vi "Controller.vi"(8 "error in (no error)":errorcluster) -> (0 "error out":errorcluster)   [LabVIEW 2017]
uses:
  Type Definitions/Controller Data.ctl
  Type Definitions/DB Data.ctl
  Type Definitions/DB Info.ctl
  Type Definitions/Display Data.ctl
  Type Definitions/DB Record.ctl
  Type Definitions/Display Console States.ctl
  Type Definitions/GUI Data.ctl
  Type Definitions/Controller States.ctl
  Type Definitions/Sensor UI Data.ctl
  Type Definitions/Queue FG Options.ctl
  Type Definitions/Display Console Message.ctl
  Type Definitions/Sensor Message.ctl
  Type Definitions/Sensor States.ctl
  Type Definitions/GUI Message.ctl
  Type Definitions/Database States.ctl
  Type Definitions/Database Message.ctl
  Type Definitions/Timer States.ctl
  Type Definitions/Controller Message.ctl
  Current State.vi
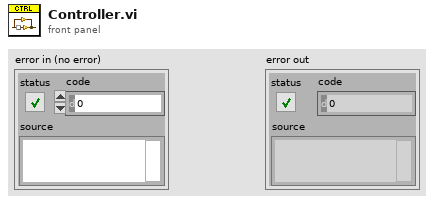
[diagram p1: front panel]
types:
  T1 = typedef "Controller Data.ctl" = cluster{"Time":dbl, "DB Data in":T2, "Display Data":T4, "GUI Data ":T7, "Sensor UI":T9, "Controller States":T8}
  T2 = typedef "DB Data.ctl" = cluster{"Account":i32, "First Name":string, "Last Name":string, "Balance":fxp<+/-,64,35>, "DB Info":T3}
  T3 = typedef "DB Info.ctl" = enum16{"Empty", "Verify", "Login Accepted", "Invalid Login", "Deposit Complete", "Withdrawal Complete", "Withdrawal Failed", "Terminate"}
  T4 = typedef "Display Data.ctl" = cluster{"Message Text":string, "DB Record":T5, "Card Read":bool, "Display Console States":T6}
  T5 = typedef "DB Record.ctl" = cluster{"Account":i32, "First Name":string, "Last Name":string, "Balance":fxp<+/-,64,35>}
  T6 = typedef "Display Console States.ctl" = enum16{"Timeout", "Initial", "Login", "Invalid Login", "Idle", "Balance Inquiry", "Deposit", "Withdrawal", "Fast Cash", "Withdrawal Failed", "Withdrawal Complete", "Terminate", "Shutdown"}
  T7 = typedef "GUI Data.ctl" = cluster{"Card Reader":enum8{"Enabled", "Disabled", "Disabled and Grayed Out"}, "Keypad":enum8{"Enabled", "Disabled", "Disabled and Grayed Out"}, "Balance Inquiry":enum8{"Enabled", "Disabled", "Disabled and Grayed Out"}, "Deposit":enum8{"Enabled", "Disabled", "Disabled and Grayed Out"}, "Withdrawal":enum8{"Enabled", "Disabled", "Disabled and Grayed Out"}, "Fast Cash":enum8{"Enabled", "Disabled", "Disabled and Grayed Out"}, "New Transaction":enum8{"Enabled", "Disabled", "Disabled and Grayed Out"}, "Terminate Session":enum8{"Enabled", "Disabled", "Disabled and Grayed Out"}, "Pinpad Value":string, "Timeout":i32, "Controller States":T8}
  T8 = typedef "Controller States.ctl" = enum16{"Timeout", "Initial", "Login", "Idle", "Balance Inquiry", "Deposit", "Withdrawal", "Fast Cash", "Terminate", "Wait on Exit", "Shutdown", "Error Handler"}
  T9 = typedef "Sensor UI Data.ctl" = cluster{"Funds dispensed":enum16{"Enabled", "Disabled", "Disabled and Grayed Out"}, "Deposit received":enum16{"Enabled", "Disabled", "Disabled and Grayed Out"}, "Timeout":dbl}
  T10 = typedef "Queue FG Options.ctl" = enum16{"Set", "Get", "Read", "Write", "Destroy"}
  T11 = enum8{"Enabled", "Disabled", "Disabled and Grayed Out"}
  T12 = typedef "GUI Message.ctl" = cluster{"Message Info":T8, "Message Data":variant}
  T13 = enum16{"Enabled", "Disabled", "Disabled and Grayed Out"}
  T14 = typedef "Sensor States.ctl" = enum16{"Initial", "Idle", "Shutdown"}
  T15 = typedef "Sensor Message.ctl" = cluster{"Message Info":T14, "Message Data":variant}
  T16 = typedef "Display Console Message.ctl" = cluster{"Message Info":T6, "Message Data":variant}
  T17 = typedef "Database Message.ctl" = cluster{"Message Info":T18, "Message Data":variant}
  T18 = typedef "Database States.ctl" = enum16{"Initial", "Verify", "Balance Inquiry", "Deposit", "Withdrawal", "Fast Cash", "Terminate", "Shutdown"}
  T19 = typedef "Timer States.ctl" = enum16{"Set", "Get"}
  T20 = typedef "Controller Message.ctl" = cluster{"Message Info":T8, "Message Data":variant}
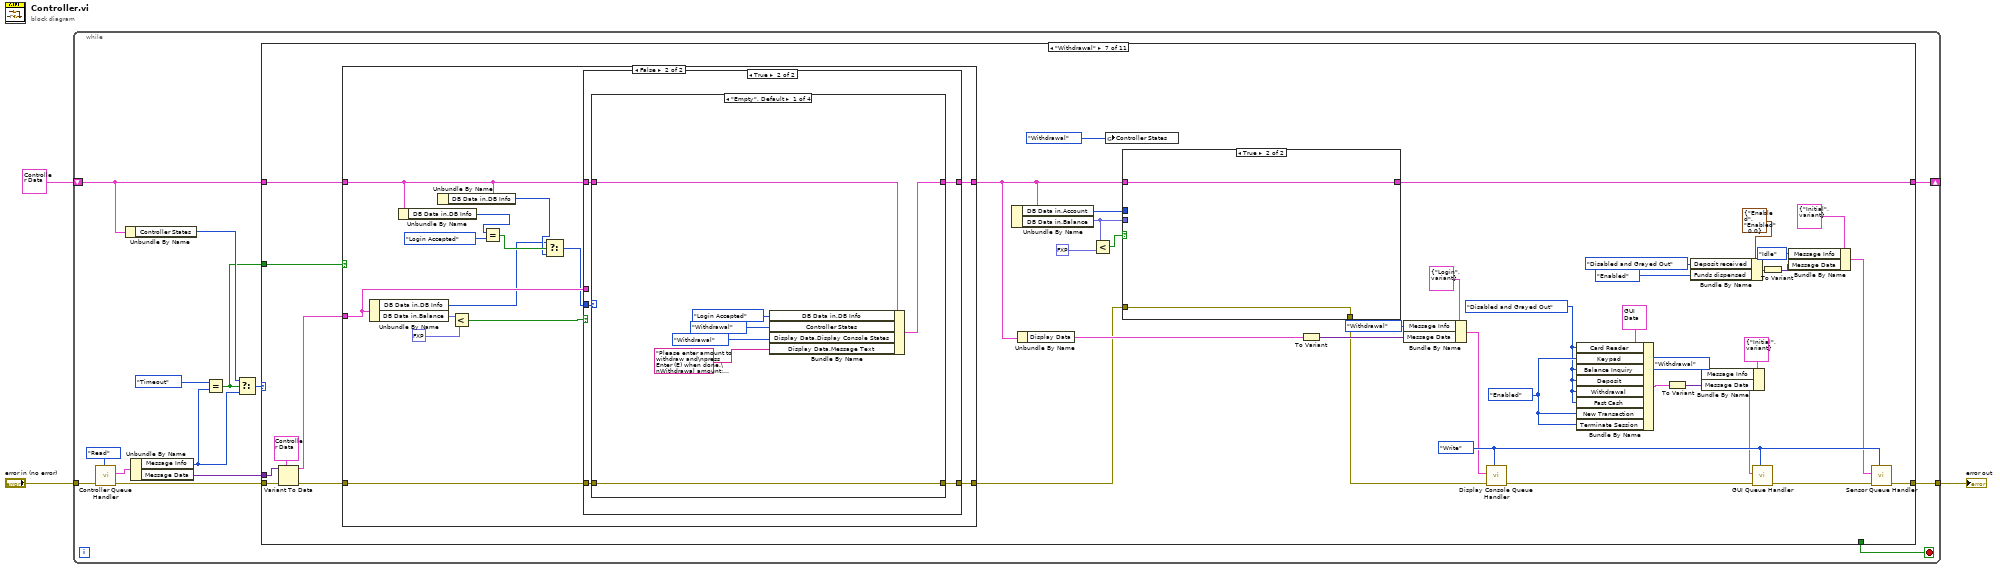
[diagram p0: block diagram]
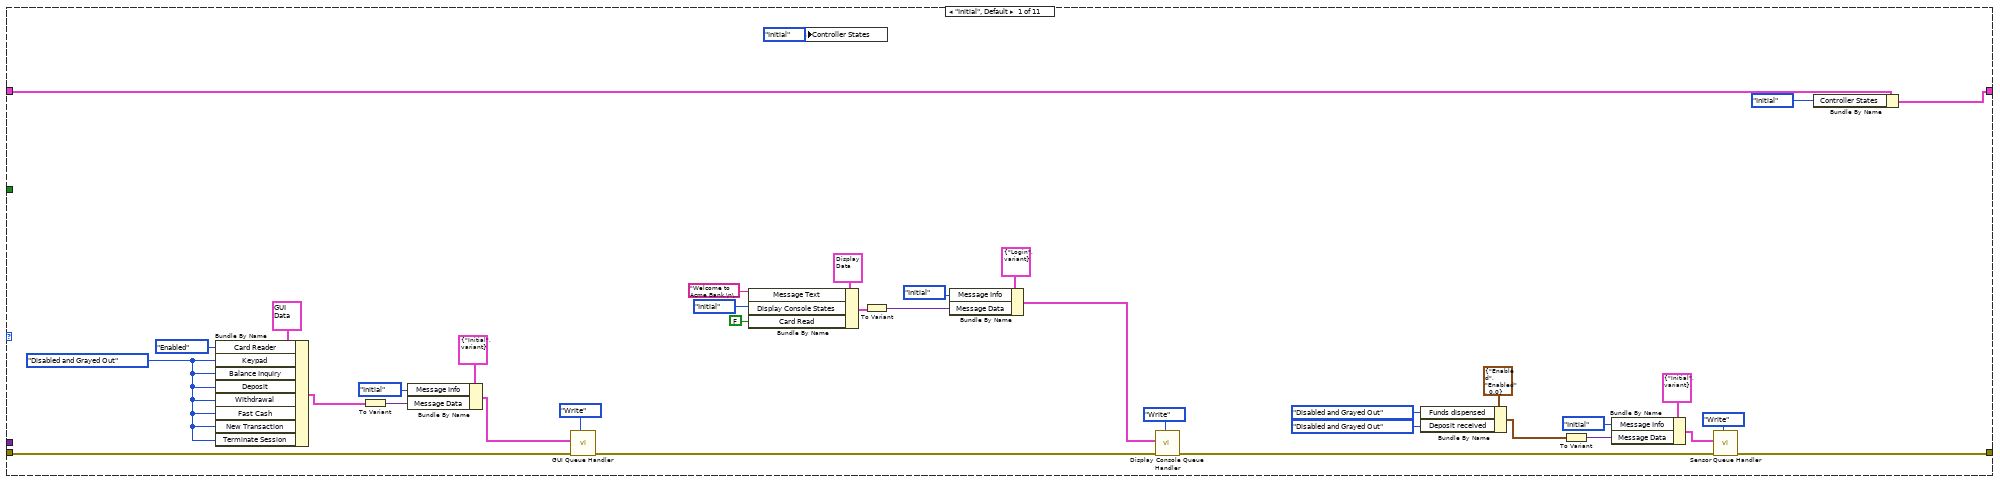
[diagram p2: hidden frame]
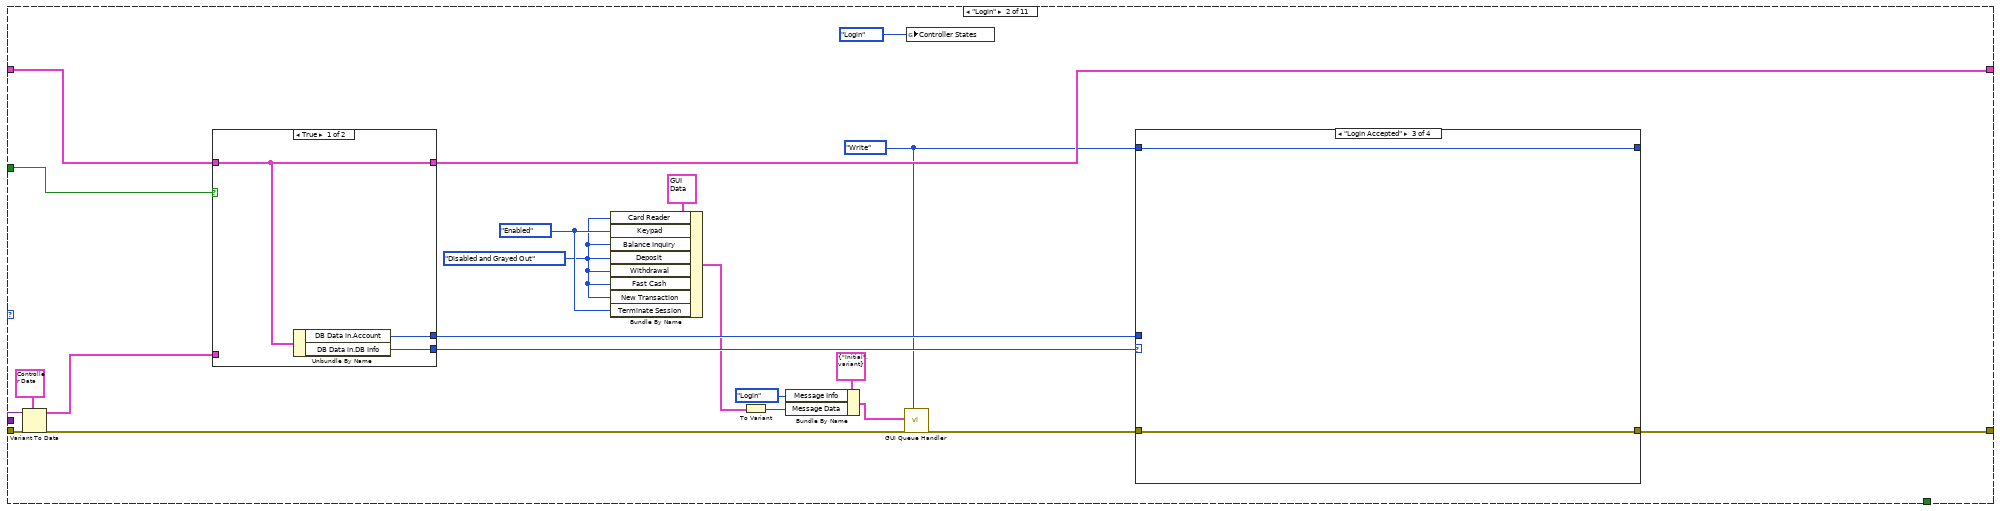
[diagram p3: hidden frame]
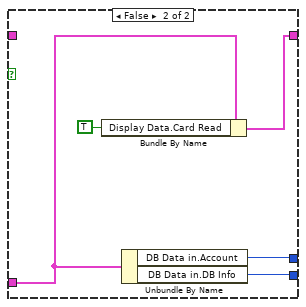
[diagram p4: hidden frame]
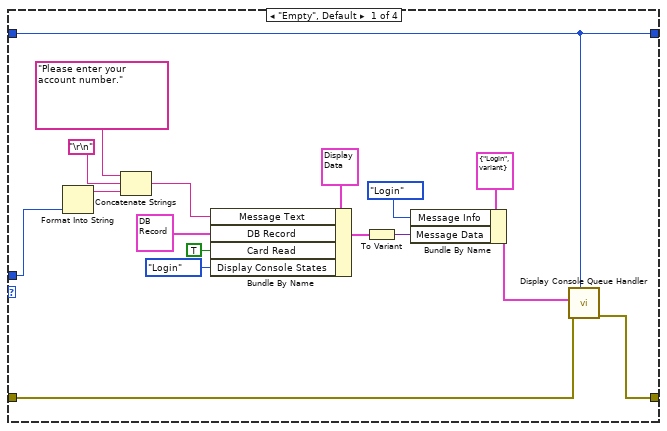
[diagram p5: hidden frame]
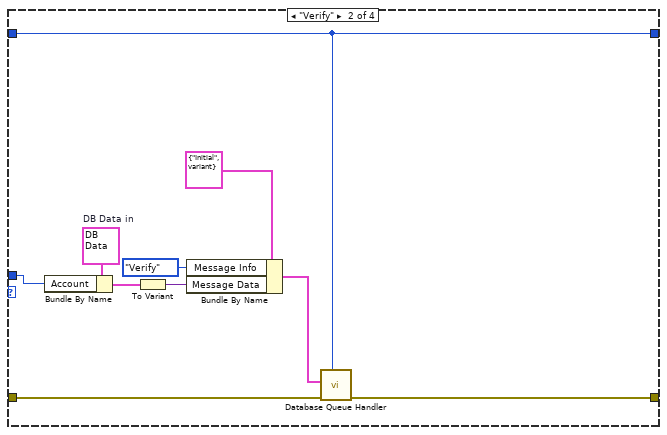
[diagram p6: hidden frame]
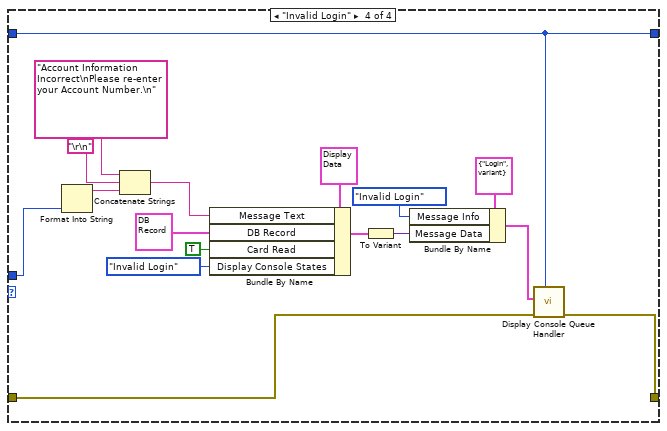
[diagram p7: hidden frame]
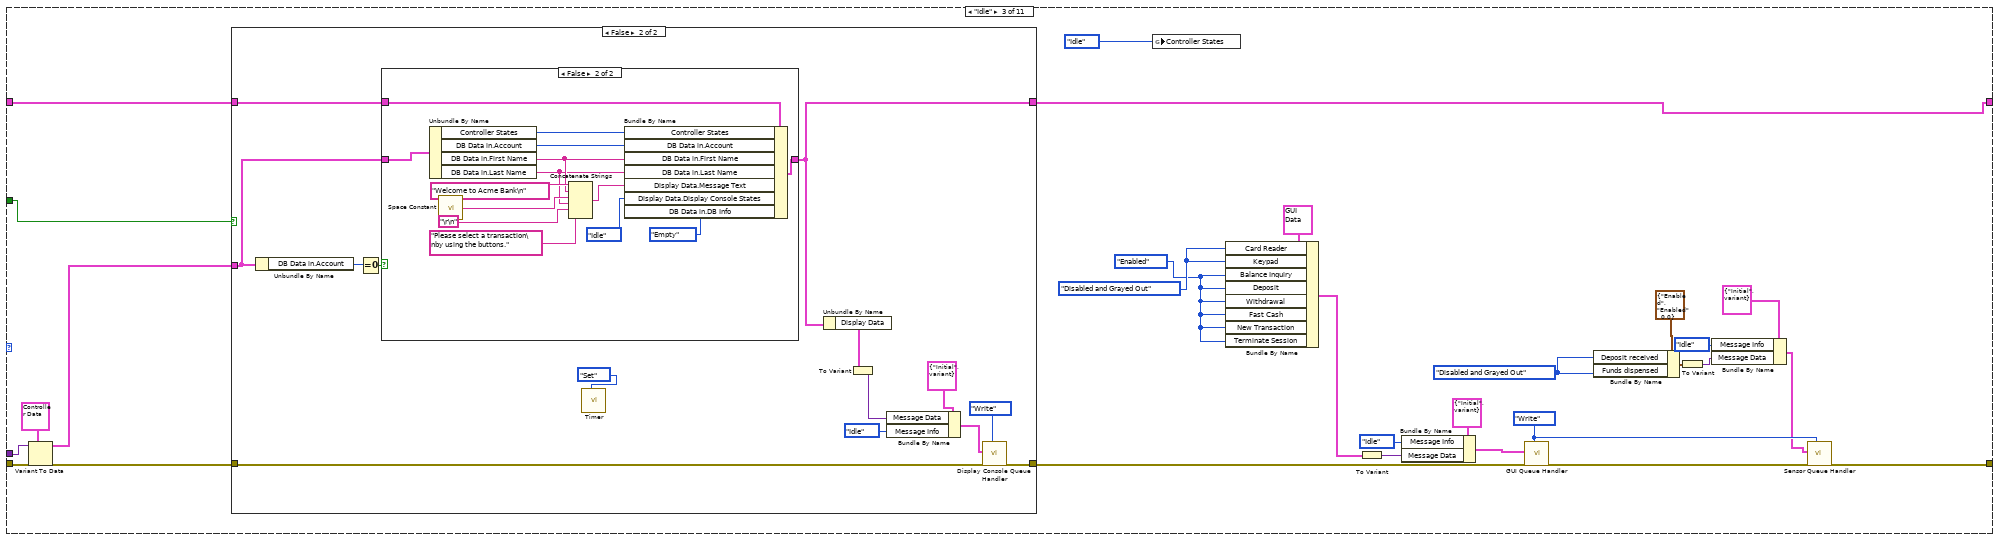
[diagram p8: hidden frame]
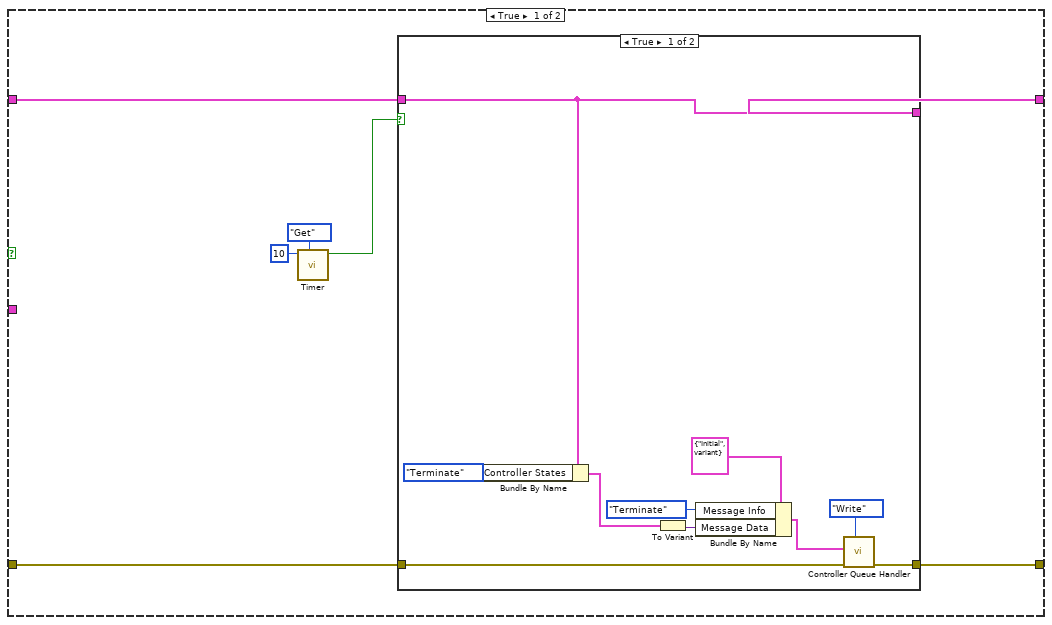
[diagram p9: hidden frame]
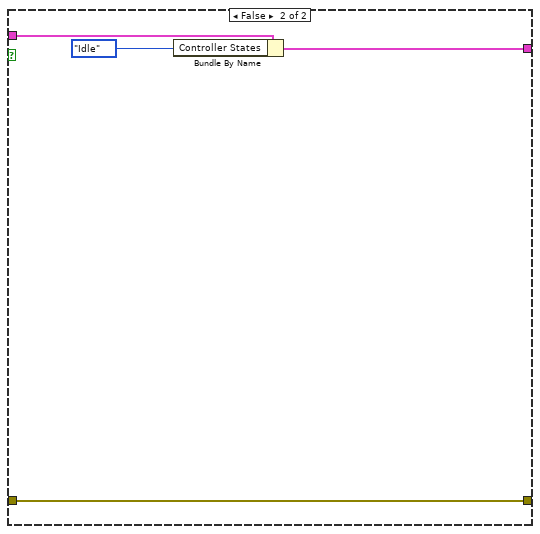
[diagram p10: hidden frame]
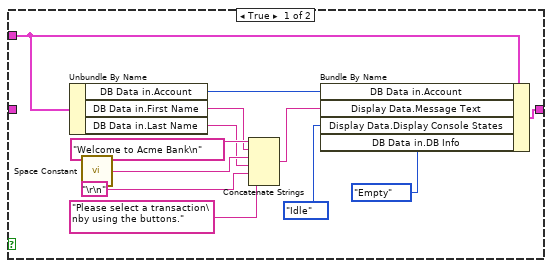
[diagram p11: hidden frame]
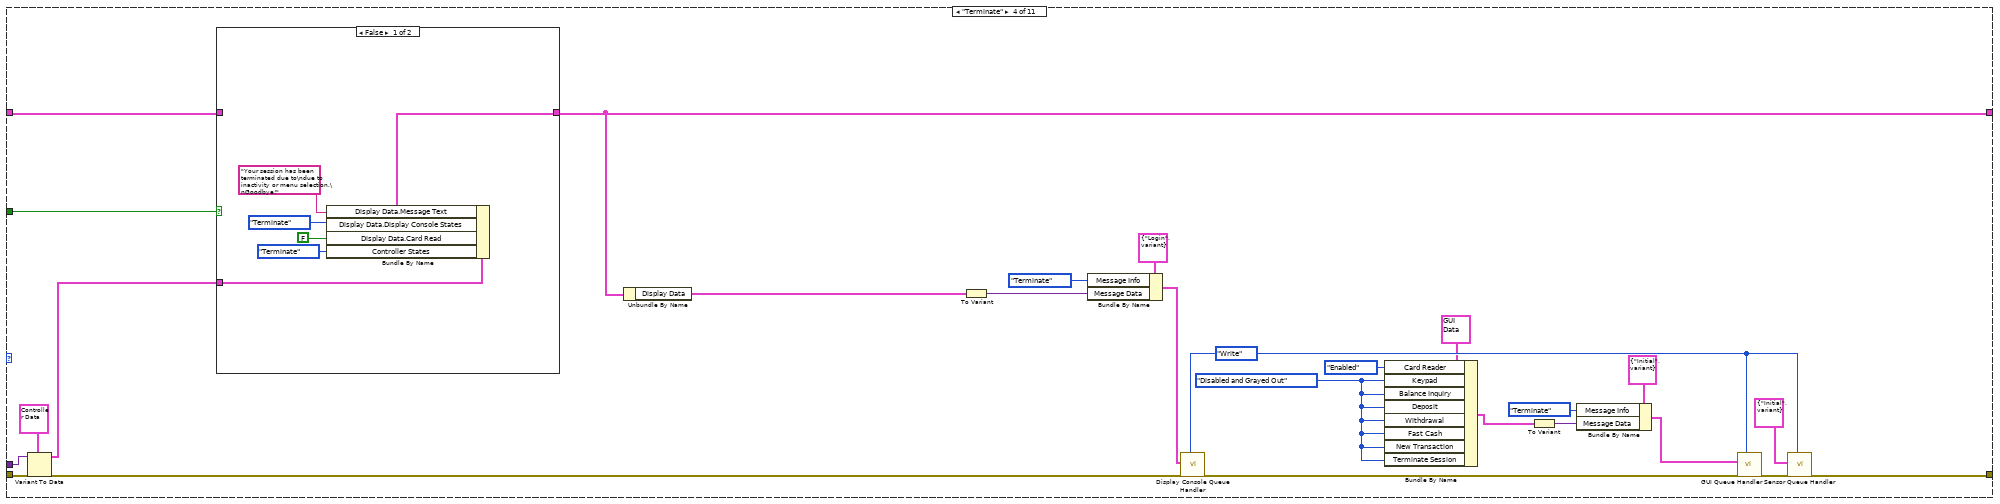
[diagram p12: hidden frame]
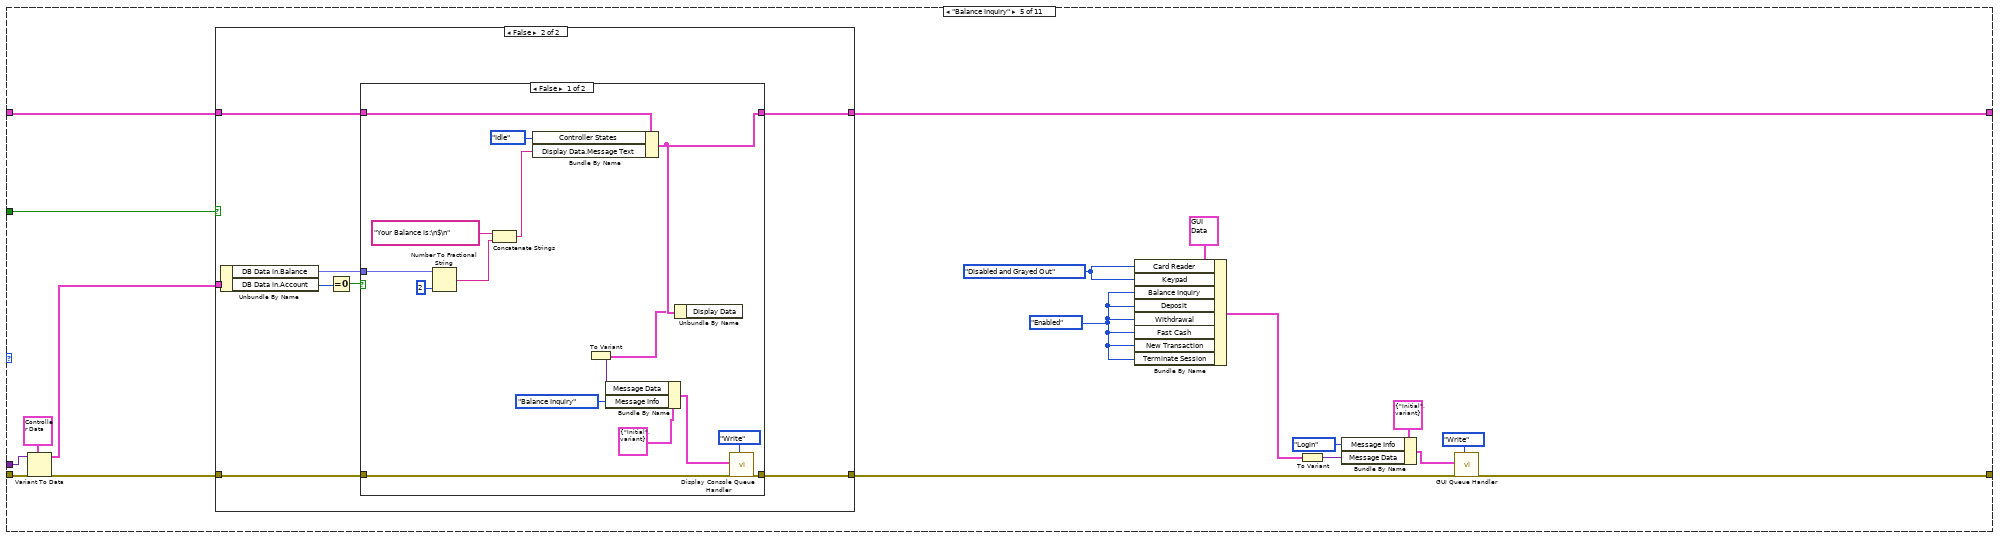
[diagram p14: hidden frame]
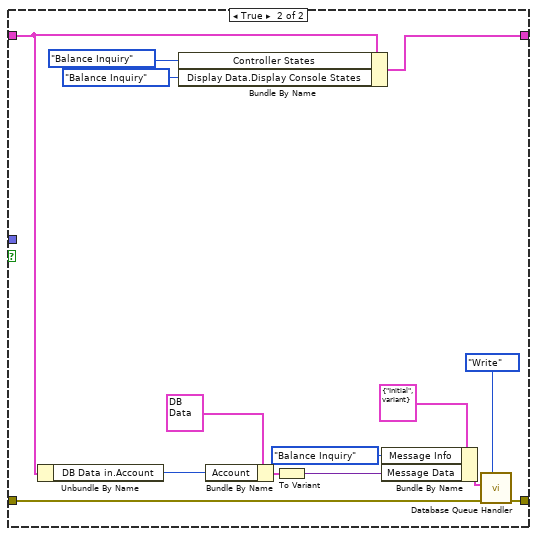
[diagram p16: hidden frame]
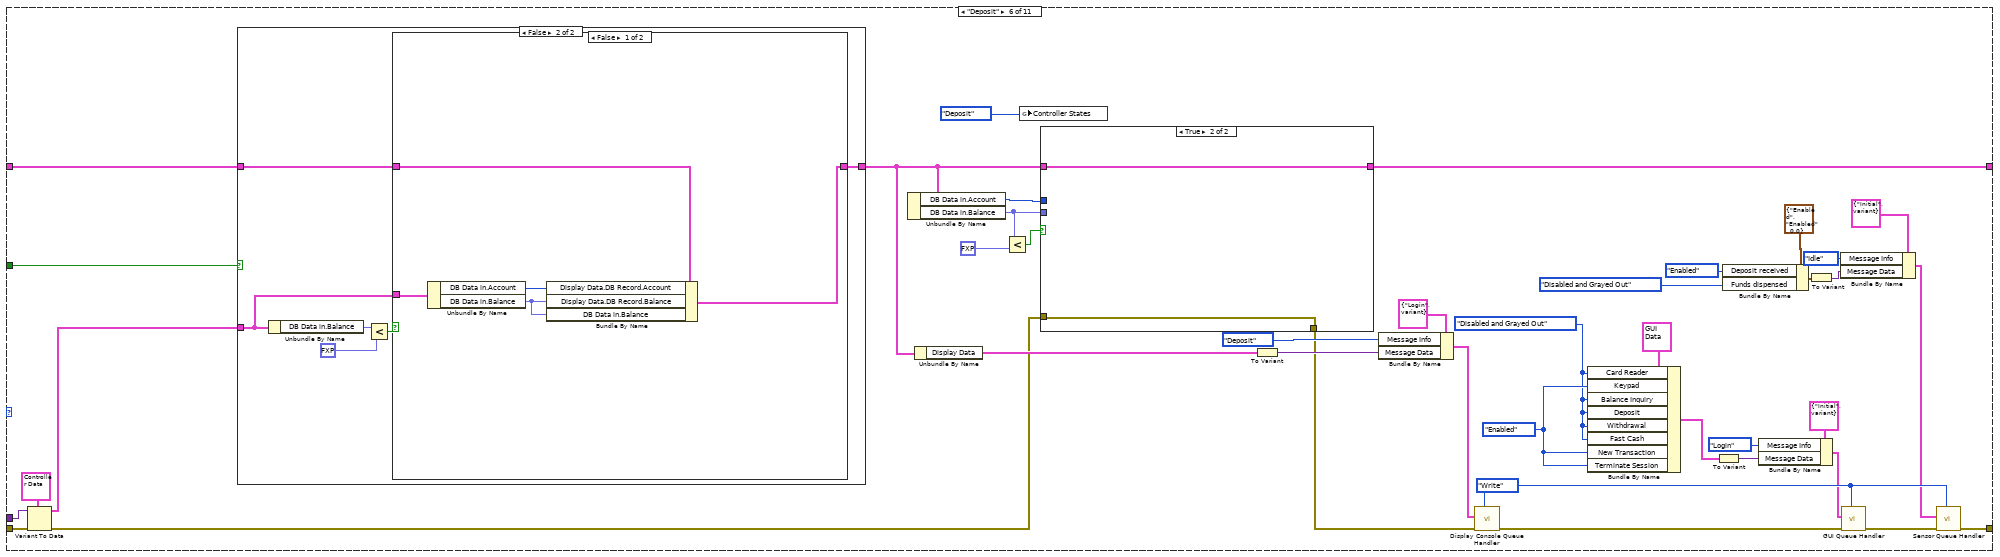
[diagram p17: hidden frame]
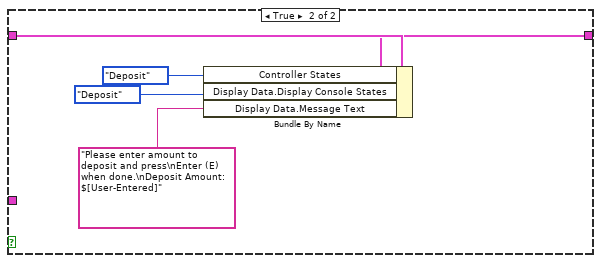
[diagram p19: hidden frame]
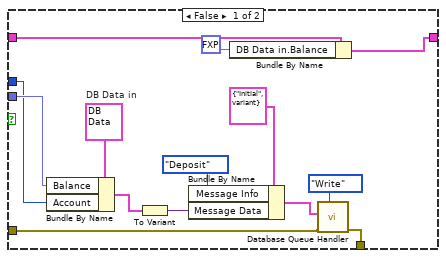
[diagram p20: hidden frame]
diagram:
  n1 = while {
    tunnel: "error in (no error)" -> [w16]
    tunnel: [w12] -> w2
    shift-right: [w10] -> _
    shift-left: T1 {"Time"=0.0, "DB Data in"={"Account"=0, "First Name"="", "Last Name"="", "Balance"=0.0, "DB Info"=enum."Login Accepted"}, "Display Data"={"Message Text"="", "DB Record"={"Account"=0, "First Name"="", "Last Name"="", "Balance"=0.0}, "Card Read"=FALSE, "Display Console States"=enum."Timeout"}, "GUI Data "={"Card Reader"=enum."Enabled", "Keypad"=enum."Enabled", "Balance Inquiry"=enum."Enabled", "Deposit"=enum."Enabled", "Withdrawal"=enum."Enabled", "Fast Cash"=enum."Enabled", "New Transaction"=enum."Enabled", "Terminate Session"=enum."Enabled", "Pinpad Value"="", "Timeout"=0, "Controller States"=enum."Initial"}, "Sensor UI"={"Funds dispensed"=enum."Enabled", "Deposit received"=enum."Enabled", "Timeout"=0.0}, "Controller States"=enum."Timeout"} ("Controller Data") -> [w6]
    stop <- w11 stop-if-true
    n2 = call "Controller Queue Handler.vi"("Action"=Queue_FG_Options."Read", "error in (no error)"=w16) -> ("error out"=w13:errorcluster, "Message out"=w15:T20)  [unwired: 7 in, 1 out]
    n3 = Unbundle By Name(w6) -> ("Controller States"=w5:T8)
    n4 = Unbundle By Name(w15) -> ("Message Info"=w7:T8, "Message Data"=w14:variant)
    n5 = Equal?(x=Controller_States."Timeout" ("Controller States"), y=w7) -> (x = y?=w4:bool)
    n6 = Select(t=w5, s=w4, f=w7) -> (s? t:f=w8:T8)
    n7 = case shown="\"Withdrawal\"" w8 {
      tunnel: w14 -> [_ w72 w156 w234 w267 w341 w415 w518 _ _ _]
      tunnel: w13 -> [w49 w75 w157 w244 w270 w350 w424 w527 w594 w621 w623]
      tunnel: [w42 w74 w134 w243 w269 w349 w423 w526 w617 w621 w623] -> w12
      tunnel: [_ _ _ _ _ _ _ _ _ TRUE _] -> w11
      tunnel: [w44 w67 w130 w229 w262 w327 w402 w505 w590 w620 w622] -> w10
      tunnel: w6 -> [w46 w69 w152 w231 w264 w338 w412 w515 w591 w620 w622]
      tunnel: w4 -> [_ w70 w154 w232 w265 w339 w413 w516 _ _ _]
      frame "Initial", Default {
        w20 = T11."Disabled and Grayed Out" ("Keypad")
        n8 = Bundle By Name(cluster=T7 {"Card Reader"=enum."Enabled", "Keypad"=enum."Enabled", "Balance Inquiry"=enum."Enabled", "Deposit"=enum."Enabled", "Withdrawal"=enum."Enabled", "Fast Cash"=enum."Enabled", "New Transaction"=enum."Enabled", "Terminate Session"=enum."Enabled", "Pinpad Value"="", "Timeout"=0, "Controller States"=enum."Initial"} ("GUI Data"), "Card Reader"=T11."Enabled", "Keypad"=w20, "Balance Inquiry"=w20, "Deposit"=w20, "Withdrawal"=w20, "Fast Cash"=w20, "New Transaction"=w20, "Terminate Session"=w20) -> (w19:T7)
        n9 = To Variant(anything=w19) -> (Variant=w18:variant)
        n10 = Bundle By Name(cluster=T12 {"Message Info"=enum."Initial", "Message Data"=variant} ("Message"), "Message Info"=Controller_States."Initial", "Message Data"=w18) -> (w24:T12)
        n11 = call "GUI Queue Handler.vi"("Action"=Queue_FG_Options."Write", "error in (no error)"=w49, "Message in"=w24) -> ("error out"=w27:errorcluster)  [unwired: 5 in, 3 out]
        n12 = Bundle By Name(cluster=T4 {"Message Text"="", "DB Record"={"Account"=0, "First Name"="", "Last Name"="", "Balance"=0.0}, "Card Read"=FALSE, "Display Console States"=enum."Timeout"} ("Display Data"), "Message Text"="Welcome to Acme Bank.\n\nPlease insert your card.", "Display Console States"=Display_Console_States."Initial", "Card Read"=FALSE) -> (w28:T4)
        n13 = global write "Current State.vi" "Controller States"(Controller_States."Initial" ("Controller States")) -> ()
        n14 = To Variant(anything=w28) -> (Variant=w53:variant)
        n15 = Bundle By Name(cluster=T16 {"Message Info"=enum."Login", "Message Data"=variant} ("Message"), "Message Info"=Display_Console_States."Initial", "Message Data"=w53) -> (w47:T16)
        n16 = call "Display Console Queue Handler.vi"("Action"=Queue_FG_Options."Write", "error in (no error)"=w27, "Message in"=w47) -> ("error out"=w48:errorcluster)  [unwired: 6 in, 2 out]
        n17 = Bundle By Name(cluster=T9 {"Funds dispensed"=enum."Enabled", "Deposit received"=enum."Enabled", "Timeout"=0.0} ("Sensor UI"), "Funds dispensed"=T13."Disabled and Grayed Out", "Deposit received"=T13."Disabled and Grayed Out") -> (w36:T9)
        n18 = To Variant(anything=w36) -> (Variant=w33:variant)
        n19 = Bundle By Name(cluster=T15 {"Message Info"=enum."Initial", "Message Data"=variant} ("Message"), "Message Info"=Sensor_States."Initial", "Message Data"=w33) -> (w38:T15)
        n20 = call "Sensor Queue Handler.vi"("Action"=Queue_FG_Options."Write", "error in (no error)"=w48, "Message in"=w38) -> ("error out"=w42:errorcluster)  [unwired: 5 in, 3 out]
        n21 = Bundle By Name(cluster=w46, "Controller States"=Controller_States."Initial") -> (w44:T1)
      }
      frame "Login" {
        w54 = T11."Disabled and Grayed Out" ("Keypad")
        w55 = T11."Enabled" ("Keypad")
        w62 = Queue_FG_Options."Write" ("Action")
        n22 = Variant To Data(error in=w75, type=T1 {"Time"=0.0, "DB Data in"={"Account"=0, "First Name"="", "Last Name"="", "Balance"=0.0, "DB Info"=enum."Login Accepted"}, "Display Data"={"Message Text"="", "DB Record"={"Account"=0, "First Name"="", "Last Name"="", "Balance"=0.0}, "Card Read"=FALSE, "Display Console States"=enum."Timeout"}, "GUI Data "={"Card Reader"=enum."Enabled", "Keypad"=enum."Enabled", "Balance Inquiry"=enum."Enabled", "Deposit"=enum."Enabled", "Withdrawal"=enum."Enabled", "Fast Cash"=enum."Enabled", "New Transaction"=enum."Enabled", "Terminate Session"=enum."Enabled", "Pinpad Value"="", "Timeout"=0, "Controller States"=enum."Initial"}, "Sensor UI"={"Funds dispensed"=enum."Enabled", "Deposit received"=enum."Enabled", "Timeout"=0.0}, "Controller States"=enum."Timeout"} ("Controller Data"), Variant=w72) -> (data=w68:T1, error out=w73:errorcluster)
        n23 = case shown="True" w70 {
          tunnel: w69 -> [w78 _]
          tunnel: w68 -> [_ w81]
          tunnel: [w78 w79] -> w67
          tunnel: [w77 w82] -> w66
          tunnel: [w76 w83] -> w65
          frame True {
            n24 = Unbundle By Name(w78) -> ("DB Data in.Account"=w76:i32, "DB Data in.DB Info"=w77:T3)
          }
          frame False {
            n25 = Bundle By Name(cluster=w81, "Display Data.Card Read"=TRUE) -> (w79:T1)
            n26 = Unbundle By Name(w81) -> ("DB Data in.Account"=w83:i32, "DB Data in.DB Info"=w82:T3)
          }
        }
        n27 = Bundle By Name(cluster=T7 {"Card Reader"=enum."Enabled", "Keypad"=enum."Enabled", "Balance Inquiry"=enum."Enabled", "Deposit"=enum."Enabled", "Withdrawal"=enum."Enabled", "Fast Cash"=enum."Enabled", "New Transaction"=enum."Enabled", "Terminate Session"=enum."Enabled", "Pinpad Value"="", "Timeout"=0, "Controller States"=enum."Initial"} ("GUI Data"), "Card Reader"=w54, "Keypad"=w55, "Balance Inquiry"=w54, "Deposit"=w54, "Withdrawal"=w54, "Fast Cash"=w54, "New Transaction"=w54, "Terminate Session"=w55) -> (w58:T7)
        n28 = To Variant(anything=w58) -> (Variant=w56:variant)
        n29 = Bundle By Name(cluster=T12 {"Message Info"=enum."Initial", "Message Data"=variant} ("Message"), "Message Info"=Controller_States."Login", "Message Data"=w56) -> (w59:T12)
        n30 = call "GUI Queue Handler.vi"("Action"=w62, "error in (no error)"=w73, "Message in"=w59) -> ("error out"=w63:errorcluster)  [unwired: 5 in, 3 out]
        n31 = global write "Current State.vi" "Controller States"(Controller_States."Login" ("Controller States")) -> ()
        n32 = case shown="\"Login Accepted\"" w66 {
          tunnel: w63 -> [w88 w110 w112 w129]
          tunnel: [w89 w103 w112 w128] -> w74
          tunnel: w62 -> [w87 w102 w111 w113]
          tunnel: [w87 w102 w111 w113] -> _
          tunnel: w65 -> [w84 w101 _ w114]
          frame "Empty", Default {
            n33 = Format Into String(w84) -> (resulting string=w100:string)  [unwired: 3 in, 1 out]
            n34 = Concatenate Strings("Please enter your account number.", "\r\n", w100) -> (w99:string)
            n35 = Bundle By Name(cluster=T4 {"Message Text"="", "DB Record"={"Account"=0, "First Name"="", "Last Name"="", "Balance"=0.0}, "Card Read"=FALSE, "Display Console States"=enum."Timeout"} ("Display Data"), "Message Text"=w99, "DB Record"=T5 {"Account"=0, "First Name"="", "Last Name"="", "Balance"=0.0}, "Card Read"=TRUE, "Display Console States"=Display_Console_States."Login") -> (w98:T4)
            n36 = To Variant(anything=w98) -> (Variant=w97:variant)
            n37 = Bundle By Name(cluster=T16 {"Message Info"=enum."Login", "Message Data"=variant} ("Message"), "Message Info"=Display_Console_States."Login", "Message Data"=w97) -> (w85:T16)
            n38 = call "Display Console Queue Handler.vi"("Action"=w87, "error in (no error)"=w88, "Message in"=w85) -> ("error out"=w89:errorcluster)  [unwired: 6 in, 2 out]
          }
          frame "Verify" {
            w109 = T2 {"Account"=0, "First Name"="", "Last Name"="", "Balance"=0.0, "DB Info"=enum."Login Accepted"}  # DB Data in
            n39 = Bundle By Name(cluster=w109, "Account"=w101) -> (w104:T2)
            n40 = To Variant(anything=w104) -> (Variant=w108:variant)
            n41 = Bundle By Name(cluster=T17 {"Message Info"=enum."Initial", "Message Data"=variant} ("Message"), "Message Info"=Database_States."Verify", "Message Data"=w108) -> (w106:T17)
            n42 = call "Database Queue Handler.vi"("Action"=w102, "error in (no error)"=w110, "Message in"=w106) -> ("error out"=w103:errorcluster)  [unwired: 6 in, 2 out]
          }
          frame "Login Accepted" {
          }
          frame "Invalid Login" {
            n43 = Format Into String(w114) -> (resulting string=w127:string)  [unwired: 3 in, 1 out]
            n44 = Concatenate Strings("Account Information Incorrect\nPlease re-enter your Account Number.\n", "\r\n", w127) -> (w126:string)
            n45 = Bundle By Name(cluster=T4 {"Message Text"="", "DB Record"={"Account"=0, "First Name"="", "Last Name"="", "Balance"=0.0}, "Card Read"=FALSE, "Display Console States"=enum."Timeout"} ("Display Data"), "Message Text"=w126, "DB Record"=T5 {"Account"=0, "First Name"="", "Last Name"="", "Balance"=0.0}, "Card Read"=TRUE, "Display Console States"=Display_Console_States."Invalid Login") -> (w125:T4)
            n46 = To Variant(anything=w125) -> (Variant=w124:variant)
            n47 = Bundle By Name(cluster=T16 {"Message Info"=enum."Login", "Message Data"=variant} ("Message"), "Message Info"=Display_Console_States."Invalid Login", "Message Data"=w124) -> (w115:T16)
            n48 = call "Display Console Queue Handler.vi"("Action"=w113, "error in (no error)"=w129, "Message in"=w115) -> ("error out"=w128:errorcluster)  [unwired: 6 in, 2 out]
          }
        }
      }
      frame "Idle" {
        w131 = T13."Disabled and Grayed Out" ("Funds dispensed")
        w142 = T11."Disabled and Grayed Out" ("Keypad")
        w141 = T11."Enabled" ("Keypad")
        w133 = Queue_FG_Options."Write" ("Action")
        n49 = Variant To Data(error in=w157, type=T1 {"Time"=0.0, "DB Data in"={"Account"=0, "First Name"="", "Last Name"="", "Balance"=0.0, "DB Info"=enum."Login Accepted"}, "Display Data"={"Message Text"="", "DB Record"={"Account"=0, "First Name"="", "Last Name"="", "Balance"=0.0}, "Card Read"=FALSE, "Display Console States"=enum."Timeout"}, "GUI Data "={"Card Reader"=enum."Enabled", "Keypad"=enum."Enabled", "Balance Inquiry"=enum."Enabled", "Deposit"=enum."Enabled", "Withdrawal"=enum."Enabled", "Fast Cash"=enum."Enabled", "New Transaction"=enum."Enabled", "Terminate Session"=enum."Enabled", "Pinpad Value"="", "Timeout"=0, "Controller States"=enum."Initial"}, "Sensor UI"={"Funds dispensed"=enum."Enabled", "Deposit received"=enum."Enabled", "Timeout"=0.0}, "Controller States"=enum."Timeout"} ("Controller Data"), Variant=w156) -> (data=w153:T1, error out=w150:errorcluster)
        n50 = case shown="False" w154 {
          tunnel: w153 -> [_ w183]
          tunnel: w152 -> [w161 w192]
          tunnel: [w160 w184] -> w130
          tunnel: w150 -> [w159 w191]
          tunnel: [w158 w190] -> w149
          frame True {
            n51 = call "Timer.vi"("Timer States"=Timer_States."Get", "Time to timeout"=u32 10) -> ("Timeout"=w162:bool)  [unwired: 9 in]
            n52 = case shown="True" w162 {
              tunnel: [w167 w178] -> w160
              tunnel: w161 -> [w167 w176]
              tunnel: w159 -> [w174 w175]
              tunnel: [w173 w175] -> w158
              frame True {
                n53 = Bundle By Name(cluster=w167, "Controller States"=Controller_States."Terminate") -> (w165:T1)
                n54 = To Variant(anything=w165) -> (Variant=w169:variant)
                n55 = Bundle By Name(cluster=T20 {"Message Info"=enum."Initial", "Message Data"=variant} ("Message"), "Message Info"=Controller_States."Terminate", "Message Data"=w169) -> (w170:T20)
                n56 = call "Controller Queue Handler.vi"("Action"=Queue_FG_Options."Write", "error in (no error)"=w174, "Message in"=w170) -> ("error out"=w173:errorcluster)  [unwired: 6 in, 2 out]
              }
              frame False {
                n57 = Bundle By Name(cluster=w176, "Controller States"=Controller_States."Idle") -> (w178:T1)
              }
            }
          }
          frame False {
            n58 = Unbundle By Name(w183) -> ("DB Data in.Account"=w182:i32)
            n59 = Equal To 0?(x=w182) -> (x = 0?=w181:bool)
            n60 = case shown="False" w181 {
              tunnel: w192 -> [w198 w212]
              tunnel: [w202 w216] -> w184
              tunnel: w183 -> [_ w207]
              frame True {
                n61 = Unbundle By Name(w198) -> ("DB Data in.Account"=w204:i32, "DB Data in.First Name"=w197:string, "DB Data in.Last Name"=w196:string)
                n62 = call <vilib>:"Space Constant.vi"() -> ("String"=w201:string)
                n63 = Concatenate Strings("Welcome to Acme Bank\n", w197, w201, w196, "\r\n", "Please select a transaction\nby using the buttons.") -> (w195:string)
                n64 = Bundle By Name(cluster=w198, "DB Data in.Account"=w204, "Display Data.Message Text"=w195, "Display Data.Display Console States"=Display_Console_States."Idle", "DB Data in.DB Info"=DB_Info."Empty") -> (w202:T1)
              }
              frame False {
                n65 = Unbundle By Name(w207) -> ("Controller States"=w205:T8, "DB Data in.Account"=w218:i32, "DB Data in.First Name"=w211:string, "DB Data in.Last Name"=w210:string)
                n66 = call <vilib>:"Space Constant.vi"() -> ("String"=w215:string)
                n67 = Concatenate Strings("Welcome to Acme Bank\n", w211, w215, w210, "\r\n", "Please select a transaction\nby using the buttons.") -> (w209:string)
                n68 = Bundle By Name(cluster=w212, "Controller States"=w205, "DB Data in.Account"=w218, "DB Data in.First Name"=w211, "DB Data in.Last Name"=w210, "Display Data.Message Text"=w209, "Display Data.Display Console States"=Display_Console_States."Idle", "DB Data in.DB Info"=DB_Info."Empty") -> (w216:T1)
              }
            }
            n69 = call "Timer.vi"("Timer States"=Timer_States."Set") -> ()  [unwired: 10 in, 1 out]
            n70 = Unbundle By Name(w184) -> ("Display Data"=w188:T4)
            n71 = To Variant(anything=w188) -> (Variant=w180:variant)
            n72 = Bundle By Name(cluster=T16 {"Message Info"=enum."Initial", "Message Data"=variant} ("Message"), "Message Data"=w180, "Message Info"=Display_Console_States."Idle") -> (w187:T16)
            n73 = call "Display Console Queue Handler.vi"("Action"=Queue_FG_Options."Write", "error in (no error)"=w191, "Message in"=w187) -> ("error out"=w190:errorcluster)  [unwired: 6 in, 2 out]
          }
        }
        n74 = global write "Current State.vi" "Controller States"(Controller_States."Idle" ("Controller States")) -> ()
        n75 = Bundle By Name(cluster=T7 {"Card Reader"=enum."Enabled", "Keypad"=enum."Enabled", "Balance Inquiry"=enum."Enabled", "Deposit"=enum."Enabled", "Withdrawal"=enum."Enabled", "Fast Cash"=enum."Enabled", "New Transaction"=enum."Enabled", "Terminate Session"=enum."Enabled", "Pinpad Value"="", "Timeout"=0, "Controller States"=enum."Initial"} ("GUI Data"), "Card Reader"=w142, "Keypad"=w142, "Balance Inquiry"=w141, "Deposit"=w141, "Withdrawal"=w141, "Fast Cash"=w141, "New Transaction"=w141, "Terminate Session"=w141) -> (w146:T7)
        n76 = To Variant(anything=w146) -> (Variant=w144:variant)
        n77 = Bundle By Name(cluster=T12 {"Message Info"=enum."Initial", "Message Data"=variant} ("Message"), "Message Info"=Controller_States."Idle", "Message Data"=w144) -> (w143:T12)
        n78 = call "GUI Queue Handler.vi"("Action"=w133, "error in (no error)"=w149, "Message in"=w143) -> ("error out"=w135:errorcluster)  [unwired: 5 in, 3 out]
        n79 = Bundle By Name(cluster=T9 {"Funds dispensed"=enum."Enabled", "Deposit received"=enum."Enabled", "Timeout"=0.0} ("Sensor UI"), "Deposit received"=w131, "Funds dispensed"=w131) -> (w138:T9)
        n80 = To Variant(anything=w138) -> (Variant=w136:variant)
        n81 = Bundle By Name(cluster=T15 {"Message Info"=enum."Initial", "Message Data"=variant} ("Message in"), "Message Info"=Sensor_States."Idle", "Message Data"=w136) -> (w132:T15)
        n82 = call "Sensor Queue Handler.vi"("Action"=w133, "error in (no error)"=w135, "Message in"=w132) -> ("error out"=w134:errorcluster)  [unwired: 5 in, 3 out]
      }
      frame "Terminate" {
        w222 = T11."Disabled and Grayed Out" ("Keypad")
        w240 = Queue_FG_Options."Write" ("Action")
        n83 = Variant To Data(error in=w244, type=T1 {"Time"=0.0, "DB Data in"={"Account"=0, "First Name"="", "Last Name"="", "Balance"=0.0, "DB Info"=enum."Login Accepted"}, "Display Data"={"Message Text"="", "DB Record"={"Account"=0, "First Name"="", "Last Name"="", "Balance"=0.0}, "Card Read"=FALSE, "Display Console States"=enum."Timeout"}, "GUI Data "={"Card Reader"=enum."Enabled", "Keypad"=enum."Enabled", "Balance Inquiry"=enum."Enabled", "Deposit"=enum."Enabled", "Withdrawal"=enum."Enabled", "Fast Cash"=enum."Enabled", "New Transaction"=enum."Enabled", "Terminate Session"=enum."Enabled", "Pinpad Value"="", "Timeout"=0, "Controller States"=enum."Initial"}, "Sensor UI"={"Funds dispensed"=enum."Enabled", "Deposit received"=enum."Enabled", "Timeout"=0.0}, "Controller States"=enum."Timeout"} ("Controller Data"), Variant=w234) -> (data=w230:T1, error out=w235:errorcluster)
        n84 = case shown="False" w232 {
          tunnel: w231 -> [_ w251]
          tunnel: [w247 w251] -> w229
          tunnel: w230 -> [w250 _]
          frame False {
            n85 = Bundle By Name(cluster=w250, "Display Data.Message Text"="Your session has been terminated due to\ndue to inactivity or menu selection.\nGoodbye!", "Display Data.Display Console States"=Display_Console_States."Terminate", "Display Data.Card Read"=FALSE, "Controller States"=Controller_States."Terminate") -> (w247:T1)
          }
          frame True {
          }
        }
        n86 = Unbundle By Name(w229) -> ("Display Data"=w228:T4)
        n87 = To Variant(anything=w228) -> (Variant=w239:variant)
        n88 = Bundle By Name(cluster=T16 {"Message Info"=enum."Login", "Message Data"=variant} ("Message"), "Message Info"=Display_Console_States."Terminate", "Message Data"=w239) -> (w236:T16)
        n89 = call "Display Console Queue Handler.vi"("Action"=w240, "error in (no error)"=w235, "Message in"=w236) -> ("error out"=w242:errorcluster)  [unwired: 6 in, 2 out]
        n90 = Bundle By Name(cluster=T7 {"Card Reader"=enum."Enabled", "Keypad"=enum."Enabled", "Balance Inquiry"=enum."Enabled", "Deposit"=enum."Enabled", "Withdrawal"=enum."Enabled", "Fast Cash"=enum."Enabled", "New Transaction"=enum."Enabled", "Terminate Session"=enum."Enabled", "Pinpad Value"="", "Timeout"=0, "Controller States"=enum."Initial"} ("GUI Data"), "Card Reader"=T11."Enabled", "Keypad"=w222, "Balance Inquiry"=w222, "Deposit"=w222, "Withdrawal"=w222, "Fast Cash"=w222, "New Transaction"=w222, "Terminate Session"=w222) -> (w221:T7)
        n91 = To Variant(anything=w221) -> (Variant=w220:variant)
        n92 = Bundle By Name(cluster=T12 {"Message Info"=enum."Initial", "Message Data"=variant} ("Message"), "Message Info"=Controller_States."Terminate", "Message Data"=w220) -> (w219:T12)
        n93 = call "GUI Queue Handler.vi"("Action"=w240, "error in (no error)"=w242, "Message in"=w219) -> ("error out"=w241:errorcluster)  [unwired: 5 in, 3 out]
        n94 = call "Sensor Queue Handler.vi"("Action"=w240, "error in (no error)"=w241, "Message in"=T15 {"Message Info"=enum."Initial", "Message Data"=variant}) -> ("error out"=w243:errorcluster)  [unwired: 5 in, 3 out]
      }
      frame "Balance Inquiry" {
        w252 = T11."Disabled and Grayed Out" ("Keypad")
        w254 = T11."Enabled" ("Keypad")
        n95 = Variant To Data(error in=w270, type=T1 {"Time"=0.0, "DB Data in"={"Account"=0, "First Name"="", "Last Name"="", "Balance"=0.0, "DB Info"=enum."Login Accepted"}, "Display Data"={"Message Text"="", "DB Record"={"Account"=0, "First Name"="", "Last Name"="", "Balance"=0.0}, "Card Read"=FALSE, "Display Console States"=enum."Timeout"}, "GUI Data "={"Card Reader"=enum."Enabled", "Keypad"=enum."Enabled", "Balance Inquiry"=enum."Enabled", "Deposit"=enum."Enabled", "Withdrawal"=enum."Enabled", "Fast Cash"=enum."Enabled", "New Transaction"=enum."Enabled", "Terminate Session"=enum."Enabled", "Pinpad Value"="", "Timeout"=0, "Controller States"=enum."Initial"}, "Sensor UI"={"Funds dispensed"=enum."Enabled", "Deposit received"=enum."Enabled", "Timeout"=0.0}, "Controller States"=enum."Timeout"} ("Controller Data"), Variant=w267) -> (data=w263:T1, error out=w261:errorcluster)
        n96 = case shown="False" w265 {
          tunnel: w264 -> [w272 w277]
          tunnel: [w272 w280] -> w262
          tunnel: w263 -> [_ w276]
          tunnel: w261 -> [w271 w279]
          tunnel: [w271 w278] -> w260
          frame True {
          }
          frame False {
            n97 = Unbundle By Name(w276) -> ("DB Data in.Balance"=w273:fxp<+/-,64,35>, "DB Data in.Account"=w274:i32)
            n98 = Equal To 0?(x=w274) -> (x = 0?=w275:bool)
            n99 = case shown="False" w275 {
              tunnel: [w287 w310] -> w280
              tunnel: w279 -> [w296 w308]
              tunnel: [w295 w307] -> w278
              tunnel: w277 -> [w289 w306]
              tunnel: w273 -> [w290 _]
              frame False {
                n100 = Number To Fractional String(number=w290, precision (6)=i16 2) -> (F-format string=w292:string)  [unwired: 2 in]
                n101 = Concatenate Strings("Your Balance is:\n$\n", w292) -> (w288:string)
                n102 = Bundle By Name(cluster=w289, "Controller States"=Controller_States."Idle", "Display Data.Message Text"=w288) -> (w287:T1)
                n103 = Unbundle By Name(w287) -> ("Display Data"=w285:T4)
                n104 = To Variant(anything=w285) -> (Variant=w284:variant)
                n105 = Bundle By Name(cluster=T16 {"Message Info"=enum."Initial", "Message Data"=variant} ("Message"), "Message Data"=w284, "Message Info"=Display_Console_States."Balance Inquiry") -> (w282:T16)
                n106 = call "Display Console Queue Handler.vi"("Action"=Queue_FG_Options."Write", "error in (no error)"=w296, "Message in"=w282) -> ("error out"=w295:errorcluster)  [unwired: 6 in, 2 out]
              }
              frame True {
                n107 = Unbundle By Name(w306) -> ("DB Data in.Account"=w304:i32)
                n108 = Bundle By Name(cluster=w306, "Controller States"=Controller_States."Balance Inquiry", "Display Data.Display Console States"=Display_Console_States."Balance Inquiry") -> (w310:T1)
                n109 = Bundle By Name(cluster=T2 {"Account"=0, "First Name"="", "Last Name"="", "Balance"=0.0, "DB Info"=enum."Login Accepted"} ("DB Data in"), "Account"=w304) -> (w302:T2)
                n110 = To Variant(anything=w302) -> (Variant=w301:variant)
                n111 = Bundle By Name(cluster=T17 {"Message Info"=enum."Initial", "Message Data"=variant} ("Message"), "Message Info"=Database_States."Balance Inquiry", "Message Data"=w301) -> (w298:T17)
                n112 = call "Database Queue Handler.vi"("Action"=Queue_FG_Options."Write", "error in (no error)"=w308, "Message in"=w298) -> ("error out"=w307:errorcluster)  [unwired: 6 in, 2 out]
              }
            }
          }
        }
        n113 = Bundle By Name(cluster=T7 {"Card Reader"=enum."Enabled", "Keypad"=enum."Enabled", "Balance Inquiry"=enum."Enabled", "Deposit"=enum."Enabled", "Withdrawal"=enum."Enabled", "Fast Cash"=enum."Enabled", "New Transaction"=enum."Enabled", "Terminate Session"=enum."Enabled", "Pinpad Value"="", "Timeout"=0, "Controller States"=enum."Initial"} ("GUI Data"), "Card Reader"=w252, "Keypad"=w252, "Balance Inquiry"=w254, "Deposit"=w254, "Withdrawal"=w254, "Fast Cash"=w254, "New Transaction"=w254, "Terminate Session"=w254) -> (w253:T7)
        n114 = To Variant(anything=w253) -> (Variant=w257:variant)
        n115 = Bundle By Name(cluster=T12 {"Message Info"=enum."Initial", "Message Data"=variant} ("Message"), "Message Info"=Controller_States."Login", "Message Data"=w257) -> (w256:T12)
        n116 = call "GUI Queue Handler.vi"("Action"=Queue_FG_Options."Write", "error in (no error)"=w260, "Message in"=w256) -> ("error out"=w269:errorcluster)  [unwired: 5 in, 3 out]
      }
      frame "Deposit" {
        w319 = T11."Disabled and Grayed Out" ("Keypad")
        w320 = T11."Enabled" ("Keypad")
        w346 = Queue_FG_Options."Write" ("Action")
        n117 = Variant To Data(error in=w350, type=T1 {"Time"=0.0, "DB Data in"={"Account"=0, "First Name"="", "Last Name"="", "Balance"=0.0, "DB Info"=enum."Login Accepted"}, "Display Data"={"Message Text"="", "DB Record"={"Account"=0, "First Name"="", "Last Name"="", "Balance"=0.0}, "Card Read"=FALSE, "Display Console States"=enum."Timeout"}, "GUI Data "={"Card Reader"=enum."Enabled", "Keypad"=enum."Enabled", "Balance Inquiry"=enum."Enabled", "Deposit"=enum."Enabled", "Withdrawal"=enum."Enabled", "Fast Cash"=enum."Enabled", "New Transaction"=enum."Enabled", "Terminate Session"=enum."Enabled", "Pinpad Value"="", "Timeout"=0, "Controller States"=enum."Initial"}, "Sensor UI"={"Funds dispensed"=enum."Enabled", "Deposit received"=enum."Enabled", "Timeout"=0.0}, "Controller States"=enum."Timeout"} ("Controller Data"), Variant=w341) -> (data=w337:T1, error out=w330:errorcluster)
        n118 = case shown="False" w339 {
          tunnel: w338 -> [w351 w357]
          tunnel: [w351 w356] -> w328
          tunnel: w337 -> [_ w355]
          frame True {
          }
          frame False {
            n119 = Unbundle By Name(w355) -> ("DB Data in.Balance"=w354:fxp<+/-,64,35>)
            n120 = Less?(x=w354, y=fxp<+/-,64,35> 1.0) -> (x < y?=w353:bool)
            n121 = case shown="False" w353 {
              tunnel: w357 -> [w359 w367]
              tunnel: [w360 w365] -> w356
              tunnel: w355 -> [w362 _]
              frame False {
                n122 = Unbundle By Name(w362) -> ("DB Data in.Account"=w361:i32, "DB Data in.Balance"=w358:fxp<+/-,64,35>)
                n123 = Bundle By Name(cluster=w359, "Display Data.DB Record.Account"=w361, "Display Data.DB Record.Balance"=w358, "DB Data in.Balance"=w358) -> (w360:T1)
              }
              frame True {
                n124 = Bundle By Name(cluster=w367, "Controller States"=Controller_States."Deposit", "Display Data.Display Console States"=Display_Console_States."Deposit", "Display Data.Message Text"="Please enter amount to deposit and press\nEnter (E) when done.\nDeposit Amount: $[User-Entered]") -> (w365:T1)
              }
            }
          }
        }
        n125 = Unbundle By Name(w328) -> ("DB Data in.Account"=w331:i32, "DB Data in.Balance"=w332:fxp<+/-,64,35>)
        n126 = Unbundle By Name(w328) -> ("Display Data"=w336:T4)
        n127 = Less?(x=w332, y=fxp<+/-,64,35> 1.0) -> (x < y?=w333:bool)
        n128 = global write "Current State.vi" "Controller States"(Controller_States."Deposit" ("Controller States")) -> ()
        n129 = case shown="True" w333 {
          tunnel: w332 -> [w375 _]
          tunnel: w331 -> [w372 _]
          tunnel: w330 -> [w374 w383]
          tunnel: [w373 w383] -> w329
          tunnel: w328 -> [w370 w382]
          tunnel: [w368 w382] -> w327
          frame False {
            w378 = T2 {"Account"=0, "First Name"="", "Last Name"="", "Balance"=0.0, "DB Info"=enum."Login Accepted"}  # DB Data in
            n130 = Bundle By Name(cluster=w378, "Balance"=w375, "Account"=w372) -> (w379:T2)
            n131 = To Variant(anything=w379) -> (Variant=w381:variant)
            n132 = Bundle By Name(cluster=T17 {"Message Info"=enum."Initial", "Message Data"=variant} ("Message"), "Message Info"=Database_States."Deposit", "Message Data"=w381) -> (w380:T17)
            n133 = Bundle By Name(cluster=w370, "DB Data in.Balance"=fxp<+/-,64,35> 0.0) -> (w368:T1)
            n134 = call "Database Queue Handler.vi"("Action"=Queue_FG_Options."Write", "error in (no error)"=w374, "Message in"=w380) -> ("error out"=w373:errorcluster)  [unwired: 6 in, 2 out]
          }
          frame True {
          }
        }
        n135 = To Variant(anything=w336) -> (Variant=w345:variant)
        n136 = Bundle By Name(cluster=T16 {"Message Info"=enum."Login", "Message Data"=variant} ("Message"), "Message Info"=Display_Console_States."Deposit", "Message Data"=w345) -> (w342:T16)
        n137 = call "Display Console Queue Handler.vi"("Action"=w346, "error in (no error)"=w329, "Message in"=w342) -> ("error out"=w348:errorcluster)  [unwired: 6 in, 2 out]
        n138 = Bundle By Name(cluster=T7 {"Card Reader"=enum."Enabled", "Keypad"=enum."Enabled", "Balance Inquiry"=enum."Enabled", "Deposit"=enum."Enabled", "Withdrawal"=enum."Enabled", "Fast Cash"=enum."Enabled", "New Transaction"=enum."Enabled", "Terminate Session"=enum."Enabled", "Pinpad Value"="", "Timeout"=0, "Controller States"=enum."Initial"} ("GUI Data"), "Card Reader"=w319, "Keypad"=w320, "Balance Inquiry"=w319, "Deposit"=w319, "Withdrawal"=w319, "Fast Cash"=w319, "New Transaction"=w320, "Terminate Session"=w320) -> (w322:T7)
        n139 = To Variant(anything=w322) -> (Variant=w324:variant)
        n140 = Bundle By Name(cluster=T9 {"Funds dispensed"=enum."Enabled", "Deposit received"=enum."Enabled", "Timeout"=0.0} ("Sensor UI"), "Deposit received"=T13."Enabled", "Funds dispensed"=T13."Disabled and Grayed Out") -> (w315:T9)
        n141 = Bundle By Name(cluster=T12 {"Message Info"=enum."Initial", "Message Data"=variant} ("Message"), "Message Info"=Controller_States."Login", "Message Data"=w324) -> (w321:T12)
        n142 = To Variant(anything=w315) -> (Variant=w311:variant)
        n143 = Bundle By Name(cluster=T15 {"Message Info"=enum."Initial", "Message Data"=variant} ("Message in"), "Message Info"=Sensor_States."Idle", "Message Data"=w311) -> (w317:T15)
        n144 = call "GUI Queue Handler.vi"("Action"=w346, "error in (no error)"=w348, "Message in"=w321) -> ("error out"=w347:errorcluster)  [unwired: 5 in, 3 out]
        n145 = call "Sensor Queue Handler.vi"("Action"=w346, "error in (no error)"=w347, "Message in"=w317) -> ("error out"=w349:errorcluster)  [unwired: 5 in, 3 out]
      }
      frame "Withdrawal" {
        w392 = T11."Disabled and Grayed Out" ("Keypad")
        w393 = T11."Enabled" ("Keypad")
        w420 = Queue_FG_Options."Write" ("Action")
        n146 = Variant To Data(error in=w424, type=T1 {"Time"=0.0, "DB Data in"={"Account"=0, "First Name"="", "Last Name"="", "Balance"=0.0, "DB Info"=enum."Login Accepted"}, "Display Data"={"Message Text"="", "DB Record"={"Account"=0, "First Name"="", "Last Name"="", "Balance"=0.0}, "Card Read"=FALSE, "Display Console States"=enum."Timeout"}, "GUI Data "={"Card Reader"=enum."Enabled", "Keypad"=enum."Enabled", "Balance Inquiry"=enum."Enabled", "Deposit"=enum."Enabled", "Withdrawal"=enum."Enabled", "Fast Cash"=enum."Enabled", "New Transaction"=enum."Enabled", "Terminate Session"=enum."Enabled", "Pinpad Value"="", "Timeout"=0, "Controller States"=enum."Initial"}, "Sensor UI"={"Funds dispensed"=enum."Enabled", "Deposit received"=enum."Enabled", "Timeout"=0.0}, "Controller States"=enum."Timeout"} ("Controller Data"), Variant=w415) -> (data=w411:T1, error out=w401:errorcluster)
        n147 = case shown="False" w413 {
          tunnel: w412 -> [w426 w430]
          tunnel: [w426 w440] -> w403
          tunnel: w411 -> [_ w439]
          tunnel: w401 -> [w425 w435]
          tunnel: [w425 w434] -> w400
          frame True {
          }
          frame False {
            n148 = Unbundle By Name(w439) -> ("DB Data in.DB Info"=w428:T3, "DB Data in.Balance"=w438:fxp<+/-,64,35>)
            n149 = Unbundle By Name(w430) -> ("DB Data in.DB Info"=w433:T3)
            n150 = Unbundle By Name(w430) -> ("DB Data in.DB Info"=w429:T3)
            n151 = Less?(x=w438, y=fxp<+/-,64,35> 1.0) -> (x < y?=w437:bool)
            n152 = Equal?(x=w433, y=DB_Info."Login Accepted") -> (x = y?=w431:bool)
            n153 = Select(t=w428, s=w431, f=w429) -> (s? t:f=w427:T3)
            n154 = case shown="True" w437 {
              tunnel: w430 -> [w443 w450]
              tunnel: [w444 w449] -> w440
              tunnel: w439 -> [w446 _]
              tunnel: w427 -> [_ w451]
              tunnel: w435 -> [w441 w448]
              tunnel: [w441 w447] -> w434
              frame False {
                n155 = Unbundle By Name(w446) -> ("DB Data in.Account"=w445:i32, "DB Data in.Balance"=w442:fxp<+/-,64,35>)
                n156 = Bundle By Name(cluster=w443, "Display Data.DB Record.Account"=w445, "Display Data.DB Record.Balance"=w442, "DB Data in.Balance"=w442) -> (w444:T1)
              }
              frame True {
                n157 = case shown="\"Empty\", Default" w451 {
                  tunnel: w450 -> [w455 w463 w467 w469]
                  tunnel: [w454 w462 w466 w469] -> w449
                  tunnel: w448 -> [w453 w464 w468 w470]
                  tunnel: [w453 w464 w468 w470] -> w447
                  frame "Empty", Default {
                    n158 = Bundle By Name(cluster=w455, "DB Data in.DB Info"=DB_Info."Login Accepted", "Controller States"=Controller_States."Withdrawal", "Display Data.Display Console States"=Display_Console_States."Withdrawal", "Display Data.Message Text"="Please enter amount to withdraw and\npress Enter (E) when done.\nWithdrawal amount: AMOUNT XD\n") -> (w454:T1)
                  }
                  frame "Withdrawal Complete" {
                    n159 = Bundle By Name(cluster=w463, "Display Data.Message Text"="Please remove cash from the ATM", "Display Data.Display Console States"=Display_Console_States."Withdrawal Complete", "DB Data in.DB Info"=DB_Info."Withdrawal Complete") -> (w462:T1)
                  }
                  frame "Withdrawal Failed" {
                    n160 = Bundle By Name(cluster=w467, "Display Data.Message Text"="Insufficient funds in account.\nPlease check your account balance\nand try again") -> (w466:T1)
                  }
                  frame "Terminate" {
                  }
                }
              }
            }
          }
        }
        n161 = Unbundle By Name(w403) -> ("DB Data in.Account"=w405:i32, "DB Data in.Balance"=w406:fxp<+/-,64,35>)
        n162 = Unbundle By Name(w403) -> ("Display Data"=w410:T4)
        n163 = Less?(x=w406, y=fxp<+/-,64,35> 1.0) -> (x < y?=w407:bool)
        n164 = global write "Current State.vi" "Controller States"(Controller_States."Withdrawal" ("Controller States")) -> ()
        n165 = case shown="True" w407 {
          tunnel: w406 -> [w478 _]
          tunnel: w405 -> [w475 _]
          tunnel: w400 -> [w477 w486]
          tunnel: [w476 w486] -> w404
          tunnel: w403 -> [w473 w485]
          tunnel: [w471 w485] -> w402
          frame False {
            w481 = T2 {"Account"=0, "First Name"="", "Last Name"="", "Balance"=0.0, "DB Info"=enum."Login Accepted"}  # DB Data in
            n166 = Bundle By Name(cluster=w481, "Balance"=w478, "Account"=w475) -> (w482:T2)
            n167 = To Variant(anything=w482) -> (Variant=w484:variant)
            n168 = Bundle By Name(cluster=T17 {"Message Info"=enum."Initial", "Message Data"=variant} ("Message"), "Message Info"=Database_States."Withdrawal", "Message Data"=w484) -> (w483:T17)
            n169 = Bundle By Name(cluster=w473, "DB Data in.Balance"=fxp<+/-,64,35> 0.0) -> (w471:T1)
            n170 = call "Database Queue Handler.vi"("Action"=Queue_FG_Options."Write", "error in (no error)"=w477, "Message in"=w483) -> ("error out"=w476:errorcluster)  [unwired: 6 in, 2 out]
          }
          frame True {
          }
        }
        n171 = To Variant(anything=w410) -> (Variant=w419:variant)
        n172 = Bundle By Name(cluster=T16 {"Message Info"=enum."Login", "Message Data"=variant} ("Message"), "Message Info"=Display_Console_States."Withdrawal", "Message Data"=w419) -> (w416:T16)
        n173 = call "Display Console Queue Handler.vi"("Action"=w420, "error in (no error)"=w404, "Message in"=w416) -> ("error out"=w422:errorcluster)  [unwired: 6 in, 2 out]
        n174 = Bundle By Name(cluster=T7 {"Card Reader"=enum."Enabled", "Keypad"=enum."Enabled", "Balance Inquiry"=enum."Enabled", "Deposit"=enum."Enabled", "Withdrawal"=enum."Enabled", "Fast Cash"=enum."Enabled", "New Transaction"=enum."Enabled", "Terminate Session"=enum."Enabled", "Pinpad Value"="", "Timeout"=0, "Controller States"=enum."Initial"} ("GUI Data"), "Card Reader"=w392, "Keypad"=w393, "Balance Inquiry"=w392, "Deposit"=w392, "Withdrawal"=w392, "Fast Cash"=w392, "New Transaction"=w393, "Terminate Session"=w393) -> (w395:T7)
        n175 = To Variant(anything=w395) -> (Variant=w397:variant)
        n176 = Bundle By Name(cluster=T9 {"Funds dispensed"=enum."Enabled", "Deposit received"=enum."Enabled", "Timeout"=0.0} ("Sensor UI"), "Deposit received"=T13."Disabled and Grayed Out", "Funds dispensed"=T13."Enabled") -> (w390:T9)
        n177 = Bundle By Name(cluster=T12 {"Message Info"=enum."Initial", "Message Data"=variant} ("Message"), "Message Info"=Controller_States."Withdrawal", "Message Data"=w397) -> (w394:T12)
        n178 = call "GUI Queue Handler.vi"("Action"=w420, "error in (no error)"=w422, "Message in"=w394) -> ("error out"=w421:errorcluster)  [unwired: 5 in, 3 out]
        n179 = To Variant(anything=w390) -> (Variant=w391:variant)
        n180 = Bundle By Name(cluster=T15 {"Message Info"=enum."Initial", "Message Data"=variant} ("Message in"), "Message Info"=Sensor_States."Idle", "Message Data"=w391) -> (w384:T15)
        n181 = call "Sensor Queue Handler.vi"("Action"=w420, "error in (no error)"=w421, "Message in"=w384) -> ("error out"=w423:errorcluster)  [unwired: 5 in, 3 out]
      }
      frame "Fast Cash" {
        w496 = T11."Disabled and Grayed Out" ("Keypad")
        w497 = T11."Enabled" ("Keypad")
        w523 = Queue_FG_Options."Write" ("Action")
        n182 = Variant To Data(error in=w527, type=T1 {"Time"=0.0, "DB Data in"={"Account"=0, "First Name"="", "Last Name"="", "Balance"=0.0, "DB Info"=enum."Login Accepted"}, "Display Data"={"Message Text"="", "DB Record"={"Account"=0, "First Name"="", "Last Name"="", "Balance"=0.0}, "Card Read"=FALSE, "Display Console States"=enum."Timeout"}, "GUI Data "={"Card Reader"=enum."Enabled", "Keypad"=enum."Enabled", "Balance Inquiry"=enum."Enabled", "Deposit"=enum."Enabled", "Withdrawal"=enum."Enabled", "Fast Cash"=enum."Enabled", "New Transaction"=enum."Enabled", "Terminate Session"=enum."Enabled", "Pinpad Value"="", "Timeout"=0, "Controller States"=enum."Initial"}, "Sensor UI"={"Funds dispensed"=enum."Enabled", "Deposit received"=enum."Enabled", "Timeout"=0.0}, "Controller States"=enum."Timeout"} ("Controller Data"), Variant=w518) -> (data=w514:T1, error out=w504:errorcluster)
        n183 = case shown="True" w516 {
          tunnel: w515 -> [w529 w533]
          tunnel: [w529 w543] -> w506
          tunnel: w514 -> [_ w542]
          tunnel: w504 -> [w528 w538]
          tunnel: [w528 w537] -> w503
          frame True {
          }
          frame False {
            n184 = Unbundle By Name(w542) -> ("DB Data in.DB Info"=w531:T3, "DB Data in.Balance"=w541:fxp<+/-,64,35>)
            n185 = Unbundle By Name(w533) -> ("DB Data in.DB Info"=w536:T3)
            n186 = Unbundle By Name(w533) -> ("DB Data in.DB Info"=w532:T3)
            n187 = Less?(x=w541, y=fxp<+/-,64,35> 1.0) -> (x < y?=w540:bool)
            n188 = Equal?(x=w536, y=DB_Info."Login Accepted") -> (x = y?=w534:bool)
            n189 = Select(t=w531, s=w534, f=w532) -> (s? t:f=w530:T3)
            n190 = case shown="True" w540 {
              tunnel: w533 -> [w545 w552]
              tunnel: [w546 w551] -> w543
              tunnel: w542 -> [w548 _]
              tunnel: w530 -> [_ w553]
              tunnel: w538 -> [w544 w550]
              tunnel: [w544 w549] -> w537
              frame False {
                n191 = Unbundle By Name(w548) -> ("DB Data in.Account"=w547:i32)
                n192 = Bundle By Name(cluster=w545, "Display Data.DB Record.Account"=w547) -> (w546:T1)
              }
              frame True {
                n193 = case shown="\"Empty\", Default" w553 {
                  tunnel: w552 -> [w558 w566 w570 w572]
                  tunnel: [w557 w565 w569 w572] -> w551
                  tunnel: w550 -> [w556 w567 w571 w573]
                  tunnel: [w556 w567 w571 w573] -> w549
                  frame "Empty", Default {
                    n194 = Bundle By Name(cluster=w558, "DB Data in.DB Info"=DB_Info."Login Accepted", "Controller States"=Controller_States."Fast Cash", "Display Data.Display Console States"=Display_Console_States."Fast Cash", "Display Data.Message Text"="Fast Cash $50 withdrawal processing", "DB Data in.Balance"=fxp<+/-,64,35> 50.0) -> (w557:T1)
                  }
                  frame "Withdrawal Complete" {
                    n195 = Bundle By Name(cluster=w566, "Display Data.Message Text"="Please remove cash from the ATM", "Display Data.Display Console States"=Display_Console_States."Withdrawal Complete", "DB Data in.DB Info"=DB_Info."Withdrawal Complete") -> (w565:T1)
                  }
                  frame "Withdrawal Failed" {
                    n196 = Bundle By Name(cluster=w570, "Display Data.Message Text"="Insufficient funds in account.\nPlease check your account balance\nand try again") -> (w569:T1)
                  }
                  frame "Terminate" {
                  }
                }
              }
            }
          }
        }
        n197 = Unbundle By Name(w506) -> ("DB Data in.Account"=w508:i32, "DB Data in.Balance"=w509:fxp<+/-,64,35>)
        n198 = Unbundle By Name(w506) -> ("Display Data"=w513:T4)
        n199 = Less?(x=w509, y=fxp<+/-,64,35> 1.0) -> (x < y?=w510:bool)
        n200 = global write "Current State.vi" "Controller States"(Controller_States."Fast Cash" ("Controller States")) -> ()
        n201 = case shown="False" w510 {
          tunnel: w509 -> [w581 _]
          tunnel: w508 -> [w578 _]
          tunnel: w503 -> [w580 w589]
          tunnel: [w579 w589] -> w507
          tunnel: w506 -> [w576 w588]
          tunnel: [w574 w588] -> w505
          frame False {
            w584 = T2 {"Account"=0, "First Name"="", "Last Name"="", "Balance"=0.0, "DB Info"=enum."Login Accepted"}  # DB Data in
            n202 = Bundle By Name(cluster=w584, "Balance"=w581, "Account"=w578) -> (w585:T2)
            n203 = To Variant(anything=w585) -> (Variant=w587:variant)
            n204 = Bundle By Name(cluster=T17 {"Message Info"=enum."Initial", "Message Data"=variant} ("Message"), "Message Info"=Database_States."Fast Cash", "Message Data"=w587) -> (w586:T17)
            n205 = Bundle By Name(cluster=w576, "DB Data in.Balance"=fxp<+/-,64,35> 0.0) -> (w574:T1)
            n206 = call "Database Queue Handler.vi"("Action"=Queue_FG_Options."Write", "error in (no error)"=w580, "Message in"=w586) -> ("error out"=w579:errorcluster)  [unwired: 6 in, 2 out]
          }
          frame True {
          }
        }
        n207 = To Variant(anything=w513) -> (Variant=w522:variant)
        n208 = Bundle By Name(cluster=T16 {"Message Info"=enum."Login", "Message Data"=variant} ("Message"), "Message Info"=Display_Console_States."Fast Cash", "Message Data"=w522) -> (w519:T16)
        n209 = call "Display Console Queue Handler.vi"("Action"=w523, "error in (no error)"=w507, "Message in"=w519) -> ("error out"=w525:errorcluster)  [unwired: 6 in, 2 out]
        n210 = Bundle By Name(cluster=T7 {"Card Reader"=enum."Enabled", "Keypad"=enum."Enabled", "Balance Inquiry"=enum."Enabled", "Deposit"=enum."Enabled", "Withdrawal"=enum."Enabled", "Fast Cash"=enum."Enabled", "New Transaction"=enum."Enabled", "Terminate Session"=enum."Enabled", "Pinpad Value"="", "Timeout"=0, "Controller States"=enum."Initial"} ("GUI Data"), "Card Reader"=w496, "Keypad"=w497, "Balance Inquiry"=w496, "Deposit"=w496, "Withdrawal"=w496, "Fast Cash"=w496, "New Transaction"=w497, "Terminate Session"=w497) -> (w498:T7)
        n211 = To Variant(anything=w498) -> (Variant=w500:variant)
        n212 = Bundle By Name(cluster=T9 {"Funds dispensed"=enum."Enabled", "Deposit received"=enum."Enabled", "Timeout"=0.0} ("Sensor UI"), "Deposit received"=T13."Disabled and Grayed Out", "Funds dispensed"=T13."Enabled") -> (w493:T9)
        n213 = Bundle By Name(cluster=T12 {"Message Info"=enum."Initial", "Message Data"=variant} ("Message"), "Message Info"=Controller_States."Fast Cash", "Message Data"=w500) -> (w495:T12)
        n214 = To Variant(anything=w493) -> (Variant=w494:variant)
        n215 = call "GUI Queue Handler.vi"("Action"=w523, "error in (no error)"=w525, "Message in"=w495) -> ("error out"=w524:errorcluster)  [unwired: 5 in, 3 out]
        n216 = Bundle By Name(cluster=T15 {"Message Info"=enum."Initial", "Message Data"=variant} ("Message in"), "Message Info"=Sensor_States."Idle", "Message Data"=w494) -> (w487:T15)
        n217 = call "Sensor Queue Handler.vi"("Action"=w523, "error in (no error)"=w524, "Message in"=w487) -> ("error out"=w526:errorcluster)  [unwired: 5 in, 3 out]
      }
      frame "Wait on Exit" {
        w614 = T15 {"Message Info"=enum."Initial", "Message Data"=variant}  # Message
        w616 = Queue_FG_Options."Write" ("Action")
        n218 = Bundle By Name(cluster=T9 {"Funds dispensed"=enum."Enabled", "Deposit received"=enum."Enabled", "Timeout"=0.0} ("Sensor UI"), "Funds dispensed"=T13."Enabled", "Deposit received"=T13."Enabled") -> (w598:T9)
        n219 = To Variant(anything=w598) -> (Variant=w597:variant)
        n220 = Bundle By Name(cluster=w614, "Message Info"=Sensor_States."Shutdown", "Message Data"=w597) -> (w611:T15)
        n221 = call "Sensor Queue Handler.vi"("Action"=w616, "error in (no error)"=w594, "Message in"=w611) -> ("error out"=w593:errorcluster)  [unwired: 5 in, 3 out]
        n222 = Bundle By Name(cluster=T17 {"Message Info"=enum."Initial", "Message Data"=variant} ("Message"), "Message Info"=Database_States."Shutdown") -> (w612:T17)
        n223 = Bundle By Name(cluster=T4 {"Message Text"="", "DB Record"={"Account"=0, "First Name"="", "Last Name"="", "Balance"=0.0}, "Card Read"=FALSE, "Display Console States"=enum."Timeout"} ("Display Data"), "Message Text"="Your session has been terminated due to\ndue to inactivity or menu selection.\nGoodbye!", "DB Record"=T5 {"Account"=0, "First Name"="", "Last Name"="", "Balance"=0.0}, "Card Read"=FALSE, "Display Console States"=Display_Console_States."Shutdown") -> (w610:T4)
        n224 = Bundle By Name(cluster=w591, "Controller States"=Controller_States."Shutdown") -> (w590:T1)
        n225 = call "Database Queue Handler.vi"("Action"=w616, "error in (no error)"=w593, "Message in"=w612) -> ("error out"=w618:errorcluster)  [unwired: 6 in, 2 out]
        n226 = To Variant(anything=w610) -> (Variant=w609:variant)
        n227 = Bundle By Name(cluster=T16 {"Message Info"=enum."Login", "Message Data"=variant} ("Message"), "Message Info"=Display_Console_States."Shutdown", "Message Data"=w609) -> (w603:T16)
        n228 = call "Display Console Queue Handler.vi"("Action"=w616, "error in (no error)"=w618, "Message in"=w603) -> ("error out"=w617:errorcluster)  [unwired: 6 in, 2 out]
      }
      frame "Shutdown" {
      }
      frame "Error Handler" {
      }
    }
  }
  "error out" <- w2
